vi "Launcher.vi"() -> ()   [LabVIEW 2020]
uses:
  <userlib>/_NEVSTOP/Communicable State Machine(CSM)/_Support/GlobalEvent/GEvt-Convert Filter Rules - v1.0.vi
  <userlib>/_NEVSTOP/Communicable State Machine(CSM)/addons/INI-Static-Variable-Support/_Support/instances/_CSM - Read Log Filter Rules - v1.0.vi
  <userlib>/_NEVSTOP/Communicable State Machine(CSM)/_Support/GlobalEvent/LogFilter/SettingVIs/Set Global CSM Filter.vi
  <userlib>/_NEVSTOP/Communicable State Machine(CSM)/_Support/GlobalEvent/LogFilter/SettingVIs/Set Global LogType Filter.vi
  <userlib>/_NEVSTOP/Communicable State Machine(CSM)/_Support/GlobalEvent/LogFilter/SettingVIs/Set Global State Filter.vi
  <userlib>/_NEVSTOP/Communicable State Machine(CSM)/_Support/GlobalEvent/LogFilter/SettingVIs/Set CSM LogType Filter.vi
  <userlib>/_NEVSTOP/Communicable State Machine(CSM)/_Support/GlobalEvent/LogFilter/SettingVIs/Set CSM State Filter.vi
  <userlib>/_NEVSTOP/Communicable State Machine(CSM)/_Support/GlobalEvent/LogFilter/SettingVIs/Set Global StateType Filter.vi
  <userlib>/_NEVSTOP/Communicable State Machine(CSM)/_Support/GlobalEvent/LogFilter/SettingVIs/Set CSM StateType Filter.vi
  <userlib>/_NEVSTOP/Communicable State Machine(CSM)/addons/INI-Static-Variable-Support/_Support/instances/_CSM - Read File Logger Configuration - v1.0.vi
  CSMStand(Lite)/resource/global-rc-strings.vi
  <userlib>/NEVSTOP-Programming-Palette/Dialog & Interface/Fit VI window to Largest Dec_nevstop.vi
  <userlib>/_NEVSTOP/Communicable State Machine(CSM)/_Support/GlobalEvent/LogFilter/LogFilter.lvclass
  <userlib>/_NEVSTOP/Communicable State Machine(CSM)/addons/Watchdog/CSM Watchdog.lvlib
  <userlib>/_NEVSTOP/Communicable State Machine(CSM)/addons/Logger/CSM File Logger.lvlib
  <userlib>/_NEVSTOP/Communicable State Machine(CSM)/Communicable State Machine.lvlib
  <userlib>/_NEVSTOP/Communicable State Machine(CSM)/addons/INI-Static-Variable-Support/INI-Static-Variable-Support.lvlib
  CSMStand(Lite)/CSMStand-Engine(Lite).lvlib
panel:
  out "Information":string="Load \"csm\"..."
  out "CSMVersion":string="Powered By CSM, Copyright ?2025 NEVSTOP-LAB"
  out "CSMStand(version)":string="CSMStand-Lite"
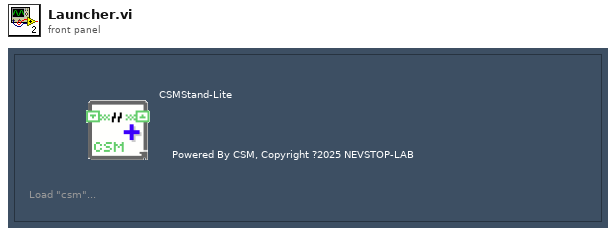
[diagram p1: front panel]
types:
  T1 = cluster{"Enable":bool, "Limit":cluster{"FileSize":i64, "FileNum":i32}, "Timestamp.Format":string, "AutoExit":bool}
  T2 = typedef "Communicable State Machine.lvlib/_CSM_GlobalLog Filter Rules - v1.0.ctl" = cluster{"Global":cluster{"CSM":string[], "LogType":T3[], "State":string[], "StateType":T4[]}, "CSM":cluster{"LogType":cluster{"CSM":string, "LogType":T3}[], "State":cluster{"CSM":string, "State":string}[], "StateType":cluster{"CSM":string, "LogType":T4}[]}}
  T3 = typedef "Communicable State Machine.lvlib/_CSM_GlobalLog_MSG_TYPE.ctl" = enum16{"User Log", "State Change", "Status", "Interrupt", "Register", "Unregister", "Error Log", "Module Created", "Module Destroyed", "Async Message", "No-Rep Async Message", "Sync Message"}
  T4 = typedef "Communicable State Machine.lvlib/_CSM_GlobalLog_STATE_TYPE.ctl" = enum16{"State - Internal State", "State - External Message", "State - Response", "State - Complete"}
  T5 = enum32{"Invalid", "Standard", "Closed", "Hidden", "Minimized", "Maximized"}
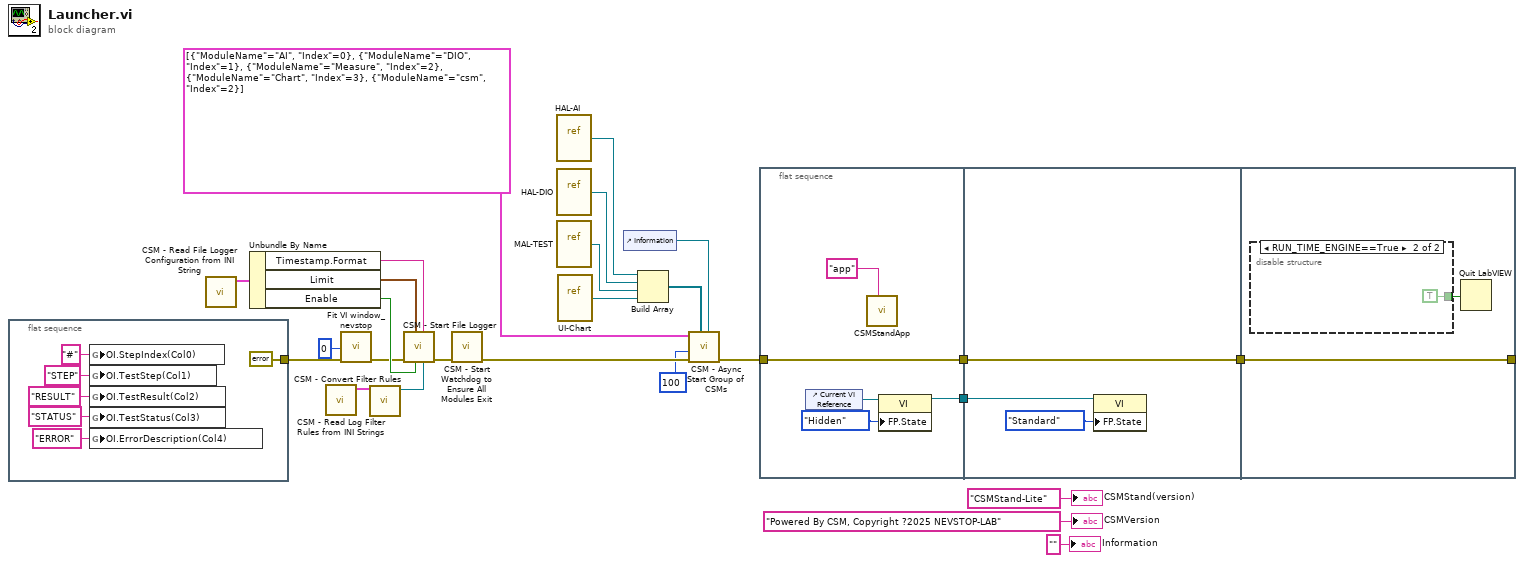
[diagram p0: block diagram]
diagram:
  n1 = flat-sequence {
    tunnel: [errorcluster {"status"=FALSE, "code"=0, "source"=""} ("error in (no error)")] -> w1
    frame #0 {
      n2 = global write "global-rc-strings.vi" "OI.StepIndex(Col0)"("#" ("OI.StepIndex(Col0)")) -> ()
      n3 = global write "global-rc-strings.vi" "OI.TestStep(Col1)"("STEP" ("OI.TestStep(Col1)")) -> ()
      n4 = global write "global-rc-strings.vi" "OI.TestResult(Col2)"("RESULT" ("OI.TestResult(Col2)")) -> ()
      n5 = global write "global-rc-strings.vi" "OI.TestStatus(Col3)"("STATUS" ("OI.TestStatus(Col3)")) -> ()
      n6 = global write "global-rc-strings.vi" "OI.ErrorDescription(Col4)"("ERROR" ("OI.TestStatus(Col3)")) -> ()
    }
  }
  n7 = call-poly <userlib>:"CSM - Read File Logger Configuration from INI String.vi"() -> ("FileLogger Configuration-v1"=w12:T1)  [unwired: 8 in, 1 out]
  n8 = Unbundle By Name(w12) -> ("Timestamp.Format"=w9:string, "Limit"=w10:cluster{"FileSize":i64, "FileNum":i32}, "Enable"=w11:bool)
  n9 = call-poly <userlib>:"CSM - Read Log Filter Rules from INI Strings.vi"() -> ("Rules-v1"=w14:T2)  [unwired: 8 in, 1 out]
  n10 = call-poly <userlib>:"Fit VI window_nevstop.vi"("error in (no error)"=w1, "border spacing (2 px)"=0) -> ("error out"=w7:errorcluster)  [unwired: 4 in, 1 out]
  n11 = call-poly <userlib>:"CSM - Convert Filter Rules.vi"("Rules-v1"=w14) -> ("GlobalLogFilter"=w15:refnum<class "LogFilter.lvclass">)  [unwired: 10 in]
  n12 = call <userlib>:"CSM - Start File Logger.vi"("Filter Rules"=w15, "Timestamp Format"=w9, "Enable? (T)"=w11, "Log Limit"=w10, "Error In"=w7) -> ("error out"=w8:errorcluster)  [unwired: 4 in, 2 out]
  n13 = call <userlib>:"CSM - Start Watchdog to Ensure All Modules Exit.vi"("error in (no error)"=w8) -> ("error out"=w23:errorcluster)  [unwired: 10 in]
  n14 = vi-ref "HAL-AI.vi"() -> (w26:refnum<vi>)
  n15 = vi-ref "HAL-DIO.vi"() -> (w25:refnum<vi>)
  n16 = vi-ref "MAL-TEST.vi"() -> (w24:refnum<vi>)
  n17 = vi-ref "UI-Chart.vi"() -> (w16:refnum<vi>)
  n18 = control-ref of="Information"() -> (w3:refnum<vi>)
  n19 = Build Array(w26, w25, w24, w16) -> (w5:refnum<vi>[])
  n20 = call "CSM - Async Start Group of CSMs.vi"("Information"=w3, "Prototypes"=w5, "error in (no error)"=w23, "interval(50ms)"=u32 100, "Module List"=cluster{"ModuleName":string, "Index":i32}[] [{"ModuleName"="AI", "Index"=0}, {"ModuleName"="DIO", "Index"=1}, {"ModuleName"="Measure", "Index"=2}, {"ModuleName"="Chart", "Index"=3}, {"ModuleName"="csm", "Index"=2}]) -> ("error out"=w21:errorcluster)  [unwired: 4 in]
  n21 = flat-sequence {
    tunnel: w21 -> [w37]
    tunnel: [w37] -> w20
    tunnel: [w34] -> w17
    tunnel: w20 -> [w40]
    tunnel: w17 -> [w38]
    tunnel: [w40] -> w13
    tunnel: [w42] -> _
    tunnel: w13 -> [w42]
    frame #0 {
      n22 = control-ref of="Current VI Reference"() -> (w36:refnum<vi>)
      n23 = call "CSMStandApp.vi"("Name(\"\" to use uuid)"="app" ("Name(\"\" to use uuid)")) -> ()  [unwired: 11 in]
      n24 = property class="VI"(reference=w36, "FP.State"=T5."Hidden" ("Front Panel Window:State")) -> (reference out=w34:refnum<vi>)  [unwired: 1 in, 1 out]
    }
    frame #1 {
      n25 = property class="VI"(reference=w38, "FP.State"=T5."Standard" ("Front Panel Window:State")) -> ()  [unwired: 1 in, 2 out]
    }
    frame #2 {
      n26 = disable-structure shown="RUN_TIME_ENGINE==True" {
        disable-tunnel: [_ TRUE ("quit? (T)")] -> w41
        frame condition #0 (active) {
        }
        frame condition #1 {
        }
      }
      n27 = Quit LabVIEW(quit? (T)=w41) -> ()
    }
  }
  "CSMStand(version)" <- "CSMStand-Lite" ("String to Prepend to Source (\"\")")
  "CSMVersion" <- "Powered By CSM, Copyright ?2025 NEVSTOP-LAB" ("String to Prepend to Source (\"\")")
  "Information" <- "" ("Information")
